vi "Align Mask and Signal - cluster.vi"(4 "Mask Selector":u16(ring) items=["ITU", "EIA/TIA 547-1989"], 6 "trigger index":i32, 8 "error in (no error)":errorcluster, 9 "lower limit":cluster{"x0":dbl, "dx":dbl, "Y":dbl[]}, 10 "upper limit":cluster{"x0":dbl, "dx":dbl, "Y":dbl[]}, 11 "Waveform":waveform(dbl)={"t0"=timestamp(0 s since 1904-01-01), "dt"=0.0, "Y"=[]}) -> (0 "error out":errorcluster, 1 "lower limit out":cluster{"x0":dbl, "dx":dbl, "Y":dbl[]}, 2 "upper limit out":cluster{"x0":dbl, "dx":dbl, "Y":dbl[]}, 3 "Waveform out":waveform(dbl), 5 "Subset Waveform":waveform(dbl))   [LabVIEW 2018]
doc: "The pulse mask tests sampled data corresponding to a quarter cycle before the trigger point. With a sampling period of 10 ns, 16 samples correspond to a quarter cycle."
uses:
  <vilib>/Waveform/WDTOps.llb/WDT Number of Waveform Samples DBL.vi
  <vilib>/Waveform/WDTOps.llb/WDT Get Waveform Subset DBL (LV80).vi
  <vilib>/Waveform/WDTOps.llb/WDT Align Waveform Timestamps DBL.vi
  <vilib>/Analysis/NI_AALBase.lvlib
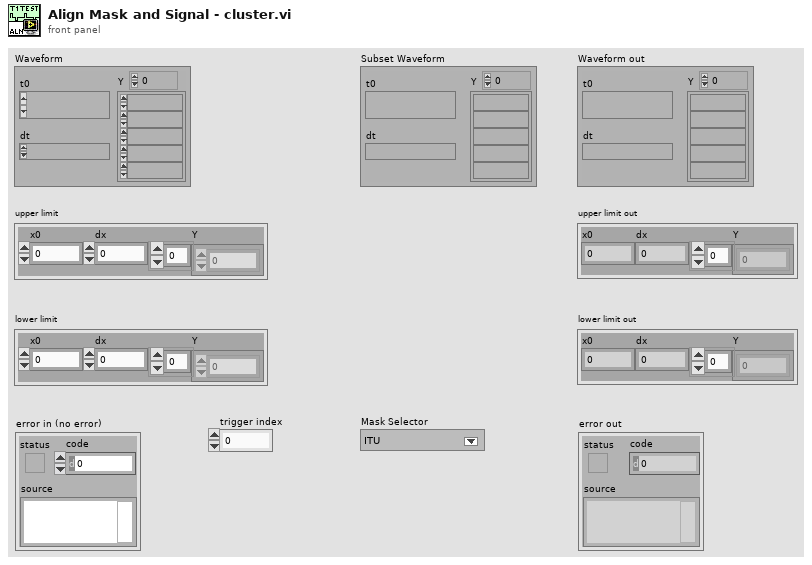
[diagram p1: front panel]
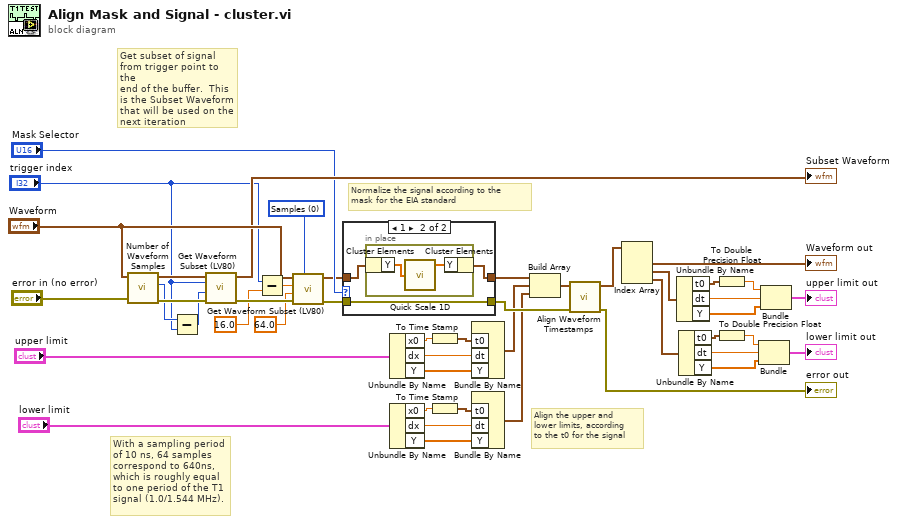
[diagram p0: block diagram]
diagram:
  w1 = u16 0 items=["Samples", "Absolute Time", "Relative Time"] ("start/duration format")
  # "Normalize the signal according to the \nmask for the EIA standard"
  # "Align the upper and \nlower limits, according \nto the t0 for the signal"
  # "With a sampling period\nof 10 ns, 64 samples\ncorrespond to 640ns, \nwhich is roughly equal \nto one period of the T1 \nsignal (1.0/1.544 MHz)."
  # "Get subset of signal\nfrom trigger point to the\nend of the buffer.  This\nis the Subset Waveform\nthat will be used on the \nnext iteration"
  n1 = call-poly <vilib>:"Number of Waveform Samples.vi"("error in (no error)"="error in (no error)", "waveform in"="Waveform") -> ("error out"=w38:errorcluster, "number of samples"=w36:i32, "waveform out"=w39:waveform(dbl))  [unwired: 7 in]
  n2 = Subtract(x=w36, y="trigger index") -> (x-y=w35:i32)
  n3 = call-poly <vilib>:"Get Waveform Subset (LV80).vi"("error in (no error)"=w38, "duration"=w35, "start samples/time"="trigger index", "waveform in"=w39) -> ("error out"=w37:errorcluster, "waveform out"=→"Subset Waveform":waveform(dbl))  [unwired: 2 in, 2 out]
  n4 = Subtract(x="trigger index", y=16.0) -> (x-y=w40:dbl)
  n5 = call-poly <vilib>:"Get Waveform Subset (LV80).vi"("start/duration format"=w1, "error in (no error)"=w37, "duration"=64.0, "start samples/time"=w40, "waveform in"="Waveform") -> ("error out"=w32:errorcluster, "waveform out"=w30:waveform(dbl))  [unwired: 1 in, 2 out]
  n6 = case shown="1" "Mask Selector" {
    tunnel: w32 -> [w48 w51]
    tunnel: [w48 w51] -> w31
    tunnel: w30 -> [w47 w50]
    tunnel: [w47 w49] -> w29
    frame Default {
    }
    frame 1 {
      n7 = in-place {
        n8 = in-place-cluster #1(w50) -> ("Y"=w52:dbl[])
        n9 = call <vilib>:"Quick Scale 1D.vi"("X"=w52) -> ("Y[i]=X[i]/Max|X|"=w53:dbl[])  [unwired: 2 out]
        n10 = in-place-cluster #1("Y"=w53) -> (w49:waveform(dbl))
      }
    }
  }
  n11 = Unbundle By Name("upper limit") -> ("x0"=w27:dbl, "dx"=w26:dbl, "Y"=w25:dbl[])
  n12 = Unbundle By Name("lower limit") -> ("x0"=w20:dbl, "dx"=w22:dbl, "Y"=w23:dbl[])
  n13 = To Time Stamp(1:w27) -> (0:w8:timestamp)
  n14 = To Time Stamp(1:w20) -> (0:w9:timestamp)
  n15 = Bundle By Name("t0"=w8, "dt"=w26, "Y"=w25) -> (w24:waveform(dbl))  [unwired: 1 in]
  n16 = Bundle By Name("t0"=w9, "dt"=w22, "Y"=w23) -> (w19:waveform(dbl))  [unwired: 1 in]
  n17 = Build Array(w29, w24, w19) -> (w44:waveform(dbl)[])
  n18 = call-poly <vilib>:"Align Waveform Timestamps.vi"("error in (no error)"=w31, "waveforms in"=w44) -> ("error out"=→"error out":errorcluster, "waveforms out"=w43:waveform(dbl)[])  [unwired: 8 in]
  n19 = Index Array(array=w43) -> (element #1=→"Waveform out":waveform(dbl), element #2=w7:waveform(dbl), element #3=w6:waveform(dbl))  [unwired: 3 in]
  n20 = Unbundle By Name(w7) -> ("t0"=w10:timestamp, "dt"=w18:dbl, "Y"=w17:dbl[])
  n21 = Unbundle By Name(w6) -> ("t0"=w11:timestamp, "dt"=w14:dbl, "Y"=w13:dbl[])
  n22 = To Double Precision Float(number=w10) -> (double precision float=w4:dbl)
  n23 = To Double Precision Float(number=w11) -> (double precision float=w15:dbl)
  n24 = Bundle(w15, "dt"=w14, "Y"=w13) -> (→"lower limit out":cluster{dbl, "dt":dbl, "Y":dbl[]})  [unwired: 1 in]
  n25 = Bundle(w4, "dt"=w18, "Y"=w17) -> (→"upper limit out":cluster{dbl, "dt":dbl, "Y":dbl[]})  [unwired: 1 in]
